vi "RSZVB Set Sweep Segment Bit Values.vi"(4 "Bit 0 (F: Off)":bool, 5 "Bit 3 (F: Off)":bool, 6 "Bit 2 (F: Off)":bool, 7 "Bit 1 (F: Off)":bool, 8 "error in (no error)":errorcluster {"code" format="%.0x"}, 9 "Segment (1)":i32=1, 10 "Channel (1)":i32=1, 11 "VISA session":refnum<visa-resource-name>) -> (0 "error out":errorcluster {"code" format="%.0x"}, 3 "dup VISA session":refnum<visa-resource-name>)   [LabVIEW 2011]
doc: "This VI sets four independent output signals at the USER CONTROL connector (lines 8, 9, 10, 11). The output signals are 3.3 V TTL signals which can be used to differentiate between up to 16 independent analyzer states for each channel.\n\nOUTPut<Ch>:UPORt:SEGMent<Seg>[:VALue]"
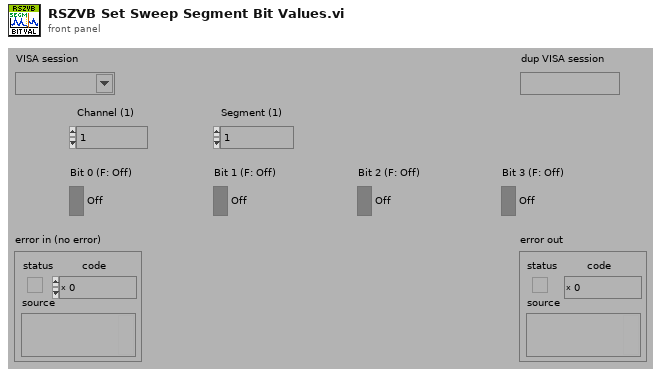
[diagram p1: front panel]
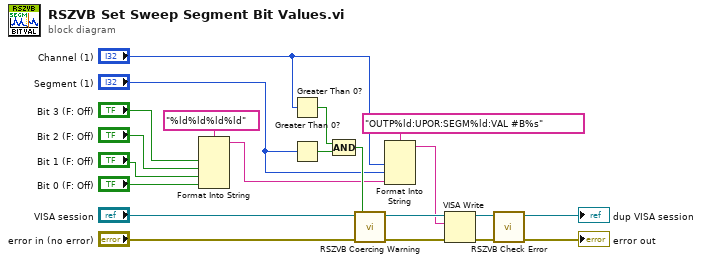
[diagram p0: block diagram]
diagram:
  n1 = Format Into String(format string="%ld%ld%ld%ld", "Bit 3 (F: Off)", "Bit 2 (F: Off)", "Bit 1 (F: Off)", "Bit 0 (F: Off)") -> (resulting string=w6:string)  [unwired: 2 in, 1 out]
  n2 = Greater Than 0?(x="Channel (1)") -> (x > 0?=w15:bool)
  n3 = Greater Than 0?(x="Segment (1)") -> (x > 0?=w14:bool)
  n4 = Compound Arithmetic op=AND(w15, w14) -> (w16:bool)
  n5 = call "RSZVB Coercing Warning.vi"("In Range?"=w16, "error in (no error)"="error in (no error)", "VISA session"="VISA session") -> ("error out"=w19:errorcluster, "dup VISA session"=w20:refnum<visa-resource-name>)  [unwired: 7 in]
  n6 = Format Into String(format string="OUTP%ld:UPOR:SEGM%ld:VAL #B%s", "Channel (1)", "Segment (1)", w6) -> (resulting string=w13:string)  [unwired: 2 in, 1 out]
  n7 = VISA Write(VISA resource name=w20, write buffer=w13, error in (no error)=w19) -> (VISA resource name out=w17:refnum<visa-resource-name>, error out=w18:errorcluster)  [unwired: 1 out]
  n8 = call "RSZVB Check Error.vi"("error in (no error)"=w18, "VISA session"=w17) -> ("error out"=→"error out":errorcluster, "dup VISA session"=→"dup VISA session":refnum<visa-resource-name>)  [unwired: 8 in]
